vi "发送.vi"() -> ()   [LabVIEW 2018]
panel:
  in  "数组 2":bool[](array[boolean])
  out "数据输出":string
  out "长度":i32
  out "连接的字符串":string
  out "数字":u32
  in  "数组":bool[](array[boolean])
  in  "数值 5":dbl
  in  "数值 4":dbl
  in  "数值 3":dbl
  in  "数值 2":dbl
  in  "数值":dbl
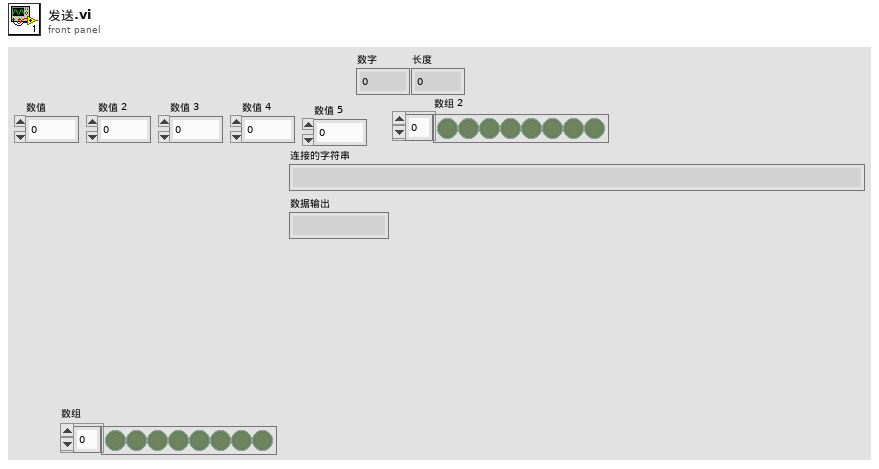
[diagram p1: front panel]
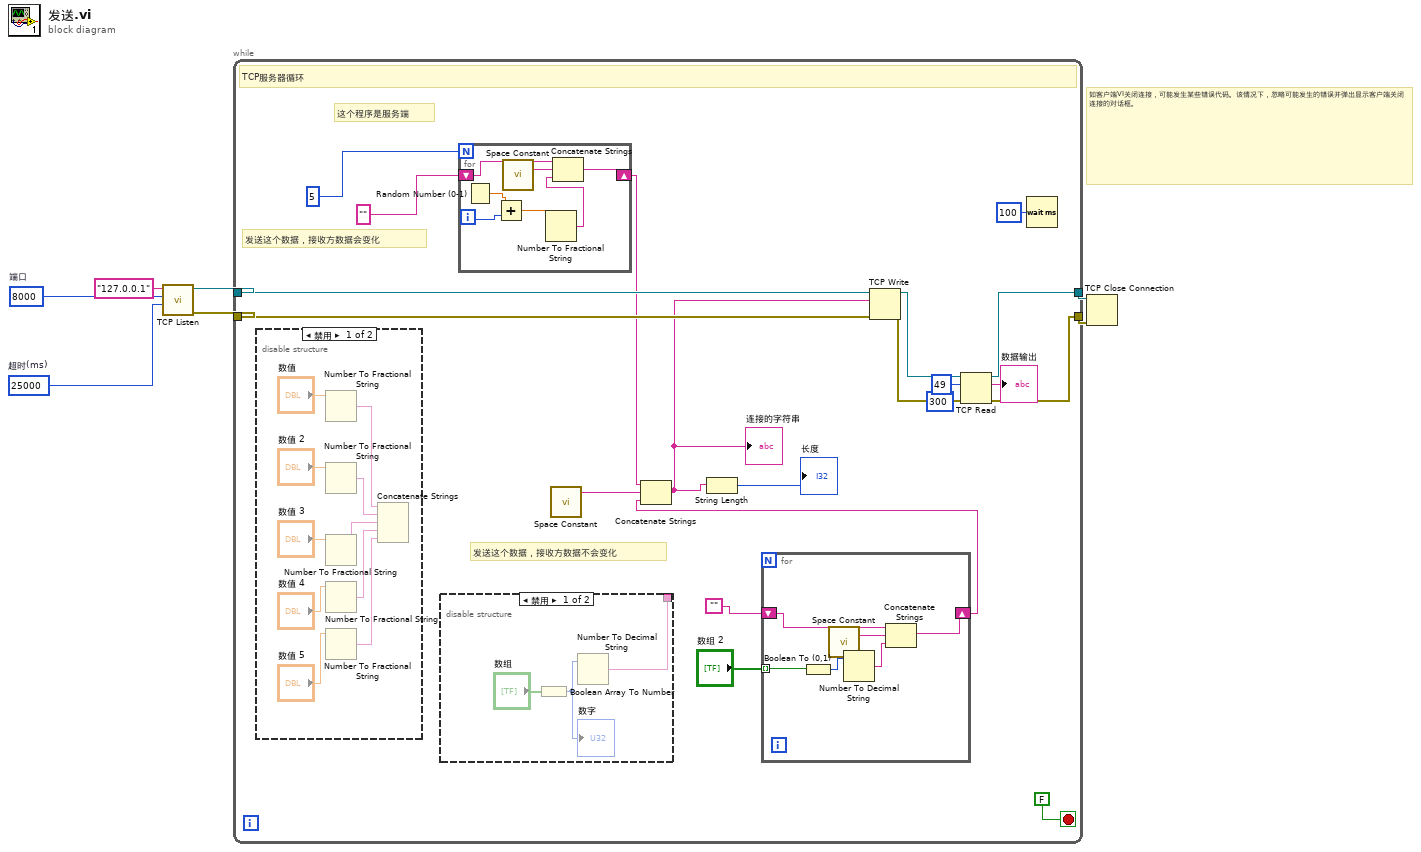
[diagram p0: block diagram]
diagram:
  w4 = u16 8000  # 端口
  w5 = 25000  # 超时(ms)
  # "如客户端VI关闭连接，可能发生某些错误代码。该情况下，忽略可能发生的错误并弹出显示客户端关闭连接的对话框。"
  n1 = call <vilib>:"TCP Listen.vi"("timeout ms (wait forever: -1)"=w5, "port"=w4, "service name"="127.0.0.1") -> ("error out"=w6:errorcluster, "connection ID"=w7:refnum<k5>)  [unwired: 4 in, 3 out]
  n2 = while {
    tunnel: w7 -> [w25]
    tunnel: w6 -> [w24]
    tunnel: [w15] -> w3
    tunnel: [w14] -> w2
    stop <- FALSE stop-if-true
    # "这个程序是服务端"
    # "发送这个数据，接收方数据会变化"
    # "发送这个数据，接收方数据不会变化"
    # "TCP服务器循环"
    n3 = disable-structure shown="禁用" {
      frame Disabled {
        n4 = Number To Fractional String(number="数值") -> (F-format string=w42:string)  [unwired: 3 in]
        n5 = Number To Fractional String(number="数值 2") -> (F-format string=w41:string)  [unwired: 3 in]
        n6 = Number To Fractional String(number="数值 3") -> (F-format string=w40:string)  [unwired: 3 in]
        n7 = Number To Fractional String(number="数值 4") -> (F-format string=w39:string)  [unwired: 3 in]
        n8 = Number To Fractional String(number="数值 5") -> (F-format string=w37:string)  [unwired: 3 in]
        n9 = Concatenate Strings(w42, w41, w40, w39, w37) -> ()  [unwired: 1 out]
      }
      frame Enabled {
      }
    }
    n10 = disable-structure shown="禁用" {
      disable-tunnel: [w34 _] -> _
      frame Disabled {
        n11 = Boolean Array To Number(Boolean array="数组") -> (number=w35:u32)
        "数字" <- w35
        n12 = Number To Decimal String(number=w35) -> (decimal integer string=w34:string)  [unwired: 1 in]
      }
      frame Enabled {
      }
    }
    n13 = for {
      N: 5 -> [_]
      shift-right: [w49] -> w18
      shift-left: "" -> [w48]
      i -> [w53]
      n14 = Random Number (0-1)() -> (number: 0 to 1=w52:dbl)
      n15 = Add(x=w52, y=w53) -> (x+y=w51:dbl)
      n16 = call <vilib>:"Space Constant.vi"() -> ("String"=w47:string)
      n17 = Number To Fractional String(number=w51) -> (F-format string=w50:string)  [unwired: 3 in]
      n18 = Concatenate Strings(w48, w47, w50) -> (w49:string)
    }
    n19 = call <vilib>:"Space Constant.vi"() -> ("String"=w22:string)
    n20 = for {
      tunnel: "数组 2" -> [w33] mode=indexing
      shift-right: [w28] -> w8
      shift-left: "" -> [w31]
      n21 = Boolean To (0,1)(Boolean=w33) -> (0, 1=w32:i16)
      n22 = call <vilib>:"Space Constant.vi"() -> ("String"=w29:string)
      n23 = Number To Decimal String(number=w32) -> (decimal integer string=w30:string)  [unwired: 1 in]
      n24 = Concatenate Strings(w31, w29, w30) -> (w28:string)
    }
    n25 = Concatenate Strings(w18, w22, w8) -> (w20:string)
    "连接的字符串" <- w20
    n26 = String Length(string=w20) -> (length=→"长度":i32)
    n27 = TCP Write(connection ID=w25, data in=w20, error in (no error)=w24) -> (connection ID out=w17:refnum<k5>, error out=w16:errorcluster)  [unwired: 2 out]
    n28 = TCP Read(connection ID=w17, bytes to read=49 ("读取的字节"), error in (no error)=w16, 9:300 ("超时毫秒(25000)")) -> (connection ID out=w15:refnum<k5>, data out=→"数据输出":string, error out=w14:errorcluster)  [unwired: 1 in]
    n29 = Wait (ms)(milliseconds to wait=u32 100) -> ()  [unwired: 1 out]
  }
  n30 = TCP Close Connection(connection ID=w3, error in (no error)=w2) -> ()  [unwired: 3 out]
